vi "DAQarm.vi"(8 "error in (no error)":errorcluster, 11 "DAQdevice in":refnum<class "DAQdevice.lvclass">) -> (0 "error out":errorcluster, 3 "DAQdevice out":refnum<class "DAQdevice.lvclass">)   [LabVIEW 2016, in "DAQdevice.lvclass"]
uses:
  DAQdevice.lvclass
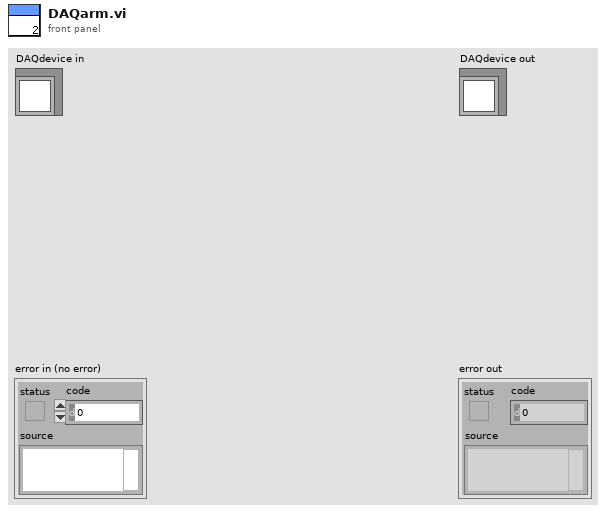
[diagram p1: front panel]
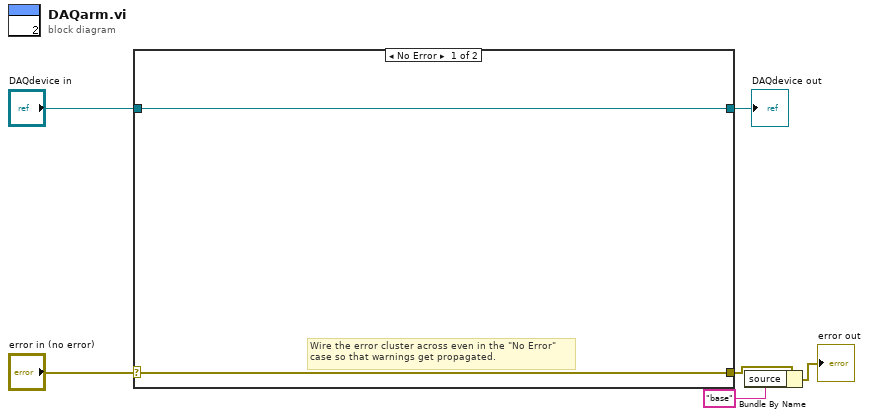
[diagram p0: block diagram]
diagram:
  n1 = case shown="No Error" "error in (no error)" {
    selector: "error in (no error)" -> [w7 w10]
    tunnel: [w7 w10] -> w3
    tunnel: [w8 w9] -> w4
    tunnel: "DAQdevice in" -> [w8 w9]
    frame No Error {
      # "Wire the error cluster across even in the \"No Error\"\ncase so that warnings get propagated."
    }
    frame Error {
    }
  }
  "DAQdevice out" <- w4
  n2 = Bundle By Name(cluster=w3, "source"="base") -> (→"error out":errorcluster)
